vi "ADCP_Update_Data_And_Control_Packets_For_Serial_Port_Reception.vi"(0 "ADCP In":refnum<class "ADCP.lvclass">, 5 "Processed Packet":u8[](array[numeric]), 11 "error in (no error)":errorcluster) -> (4 "ADCP out":refnum<class "ADCP.lvclass">, 6 "Packet Info":T1, 15 "error out":errorcluster)   [LabVIEW 2017, in "ADCP.lvclass"]
uses:
  ADCP.lvclass
  ADCP_Packet_Info.ctl
  ADCP.lvclass/ADCP.ctl
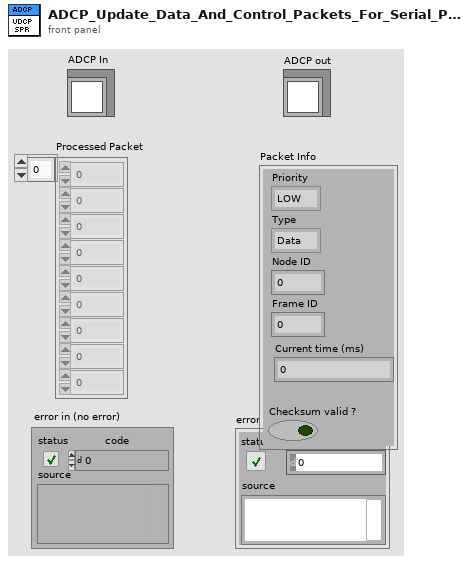
[diagram p1: front panel]
types:
  T1 = typedef "ADCP.lvclass/ADCP_Packet_Info.ctl" = cluster{"Priority":enum16{"LOW", "HIGH"}, "Type":enum16{"Data", "Connection Management", "Remote Request", "Error and status", "INVALID"}, "Node ID":i32, "Frame ID":i32, "Checksum valid ?":bool, "Current time (ms)":u32}
  T2 = enum16{"Data", "Connection Management", "Remote Request", "Error and status", "INVALID"}
  T3 = typedef "ADCP.lvclass/ADCP_Data_Packet_Transmit_Mode.ctl" = enum16{"Disable", "Single", "Cyclic", "Repeat"}
  T4 = cluster{"Parameters":cluster{"Parameter name":string, "Node name":string, "Node ID":u8, "Frame name":string, "Frame ID":u8, "Start bit":u32, "Bit length":u32, "Factor":dbl, "Offset":dbl, "Minimum":dbl, "Maximum":dbl, "Value":string, "Comments":string, "Data_Type":enum16{"BOOL", "UNSIGNED", "SIGNED", "FLOAT32", "ENUM"}, "Enum List":string[]}[], "Priority":enum16{"LOW", "HIGH"}, "Node name":string, "Node ID":u8, "Frame name":string, "Frame ID":u8, "Data":u32, "Raw bytes":u8[], "Processed bytes":u8[], "Tx count":i32, "Last Tx Time":u32, "Tx interval":u32, "Rx count":i32, "Last Rx Time":u32, "Rx interval":u32, "Tx Enable":bool, "Tx mode":T3, "Repeat/Cyclic Tx interval":u32, "Repeat count":u16}[]
  T5 = cluster{"Parameters":cluster{"Parameter name":string, "Node name":string, "Node ID":u8, "Frame name":string, "Frame ID":u8, "Start bit":u32, "Bit length":u32, "Factor":dbl, "Offset":dbl, "Minimum":dbl, "Maximum":dbl, "Value":string, "Comments":string, "Data_Type":enum16{"BOOL", "UNSIGNED", "SIGNED", "FLOAT32", "ENUM"}, "Enum List":string[]}[], "Priority":enum16{"LOW", "HIGH"}, "Node name":string, "Node ID":u8, "Frame name":string, "Frame ID":u8, "Data":u32, "Raw bytes":u8[], "Processed bytes":u8[], "Tx count":i32, "Last Tx Time":u32, "Tx interval":u32, "Rx count":i32, "Last Rx Time":u32, "Rx interval":u32, "Tx Enable":bool, "Tx mode":T3, "Repeat/Cyclic Tx interval":u32, "Repeat count":u16}
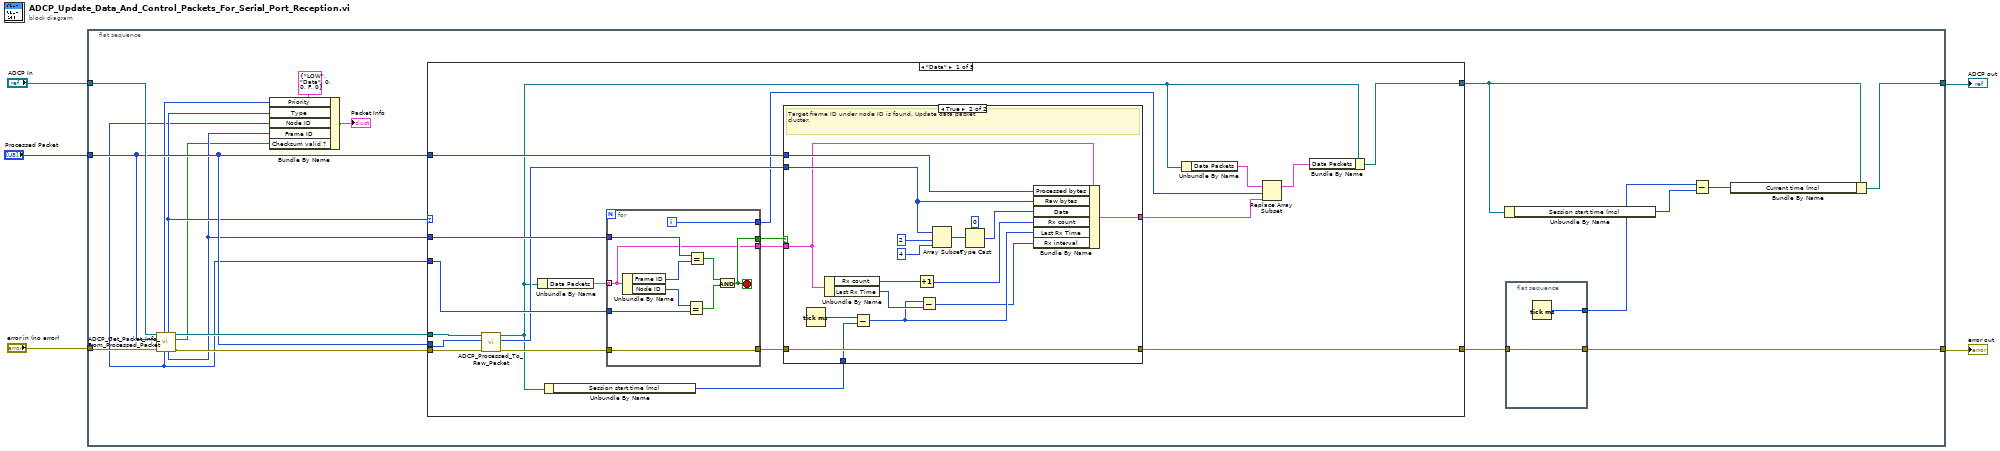
[diagram p0: block diagram]
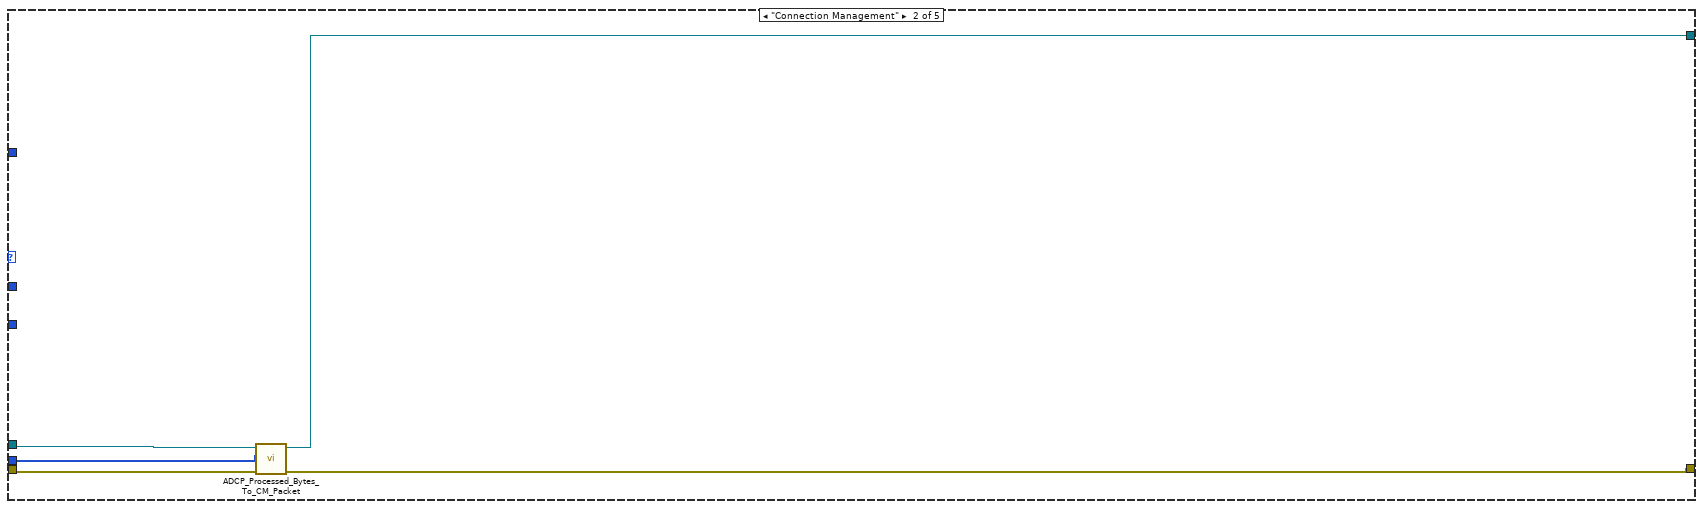
[diagram p3: hidden frame]
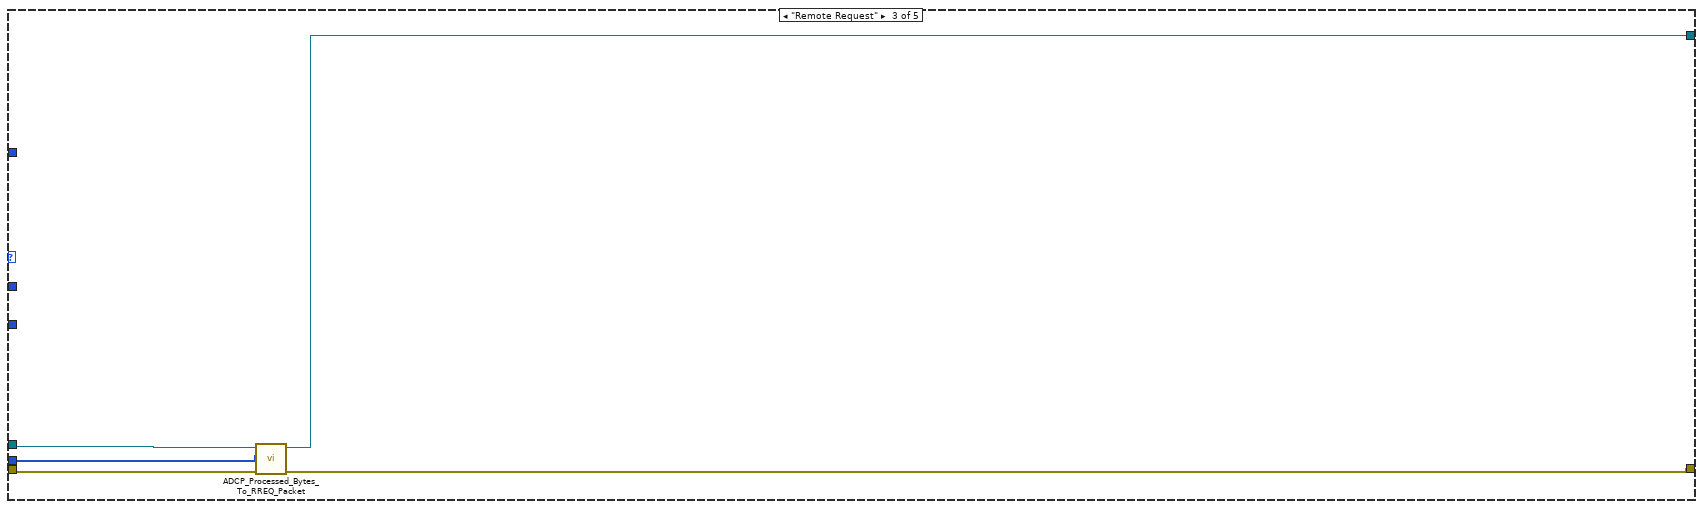
[diagram p4: hidden frame]
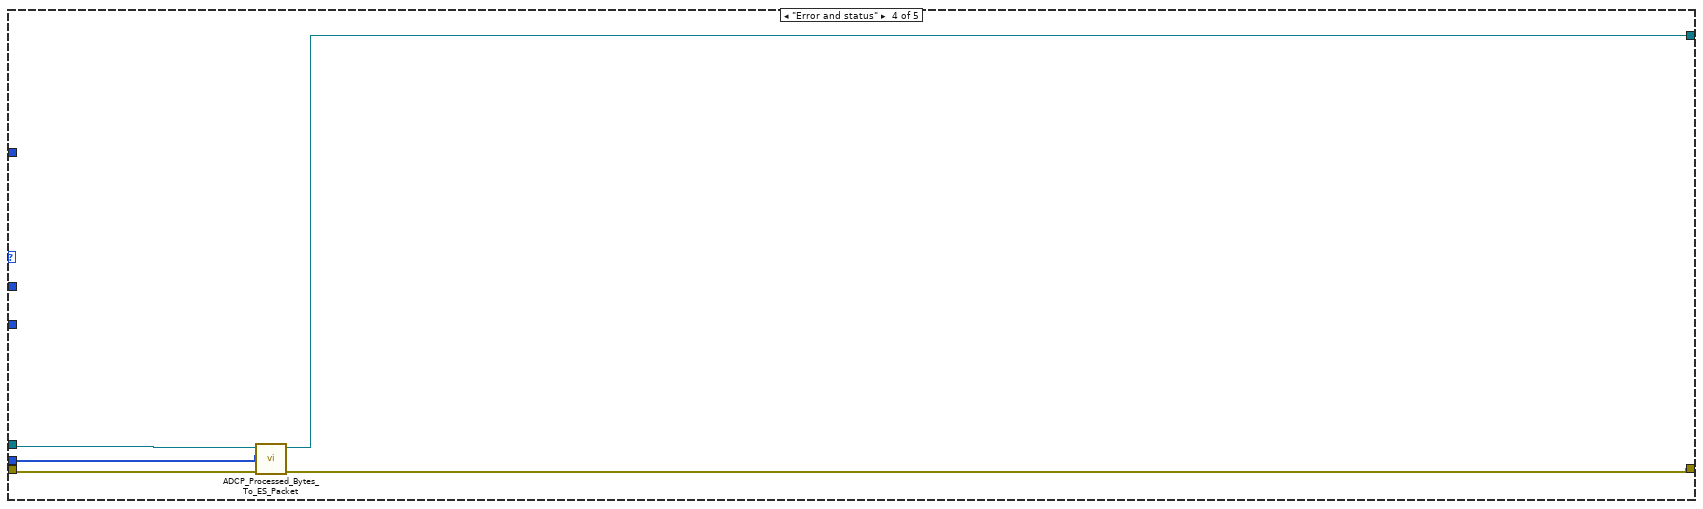
[diagram p5: hidden frame]
diagram:
  n1 = flat-sequence {
    tunnel: "ADCP In" -> [w24]
    tunnel: "Processed Packet" -> [w20]
    tunnel: "error in (no error)" -> [w23]
    tunnel: [w11] -> w1
    tunnel: [w6] -> w2
    frame #0 {
      n2 = call "ADCP_Get_Packet_Info_From_Processed_Packet.vi"("error in (no error)"=w23, "Processed Packet"=w20, "ADCP in"=w24) -> ("error out"=w22:errorcluster, "Checksum Valid ?"=w13:bool, "ADCP out"=w21:refnum<class "ADCP.lvclass">, "Packet frame ID"=w15:u8, "Packet Type"=w17:T2, "Packet node ID"=w16:u8, "Packet_Priority"=w18:enum16{"LOW", "HIGH"})  [unwired: 2 in]
      n3 = Bundle By Name(cluster=T1 {"Priority"=enum."LOW", "Type"=enum."Data", "Node ID"=0, "Frame ID"=0, "Checksum valid ?"=FALSE, "Current time (ms)"=0} ("Packet Info"), "Priority"=w18, "Type"=w17, "Node ID"=w16, "Frame ID"=w15, "Checksum valid ?"=w13) -> (→"Packet Info":T1)
      n4 = case shown="\"Data\"" w17 {
        tunnel: w22 -> [w39 w80 w85 w90 w92]
        tunnel: w21 -> [w37 w79 w84 w89 w91]
        tunnel: w20 -> [w36 w78 w83 w88 _]
        tunnel: w15 -> [w45 _ _ _ _]
        tunnel: w16 -> [w44 _ _ _ _]
        tunnel: w20 -> [w40 _ _ _ _]
        tunnel: [w30 w77 w82 w87 w92] -> w12
        tunnel: [w29 w76 w81 w86 w91] -> w8
        frame "Data" {
          n5 = call "ADCP_Processed_To_Raw_Packet.vi"("error in (no error)"=w39, "Processed Packet"=w36, "ADCP in"=w37) -> ("error out"=w38:errorcluster, "Raw Packet"=w35:u8[], "ADCP out"=w28:refnum<class "ADCP.lvclass">)  [unwired: 6 in]
          n6 = Unbundle By Name(w28) -> ("Data Packets"=w46:T4)
          n7 = Unbundle By Name(w28) -> ("Session start time (ms)"=w27:u32)
          n8 = for {
            tunnel: w38 -> [w71]
            tunnel: w46 -> [w66] mode=indexing
            tunnel: w45 -> [w75]
            tunnel: w44 -> [w72]
            tunnel: [w71] -> w42
            tunnel: [w68] -> w32
            tunnel: [w67] -> w43
            tunnel: [w66] -> w41
            i -> [w68]
            stop <- w67 stop-if-true
            n9 = Unbundle By Name(w66) -> ("Frame ID"=w74:u8, "Node ID"=w73:u8)
            n10 = Equal?(x=w73, y=w72) -> (x = y?=w69:bool)
            n11 = Equal?(x=w75, y=w74) -> (x = y?=w70:bool)
            n12 = And(x=w70, y=w69) -> (x .and. y?=w67:bool)
          }
          n13 = case shown="True" w43 {
            tunnel: w42 -> [w47 w63]
            tunnel: w41 -> [w48 w56]
            tunnel: w40 -> [_ w65]
            tunnel: w35 -> [_ w62]
            tunnel: [w48 w64] -> w33
            tunnel: [w47 w63] -> w30
            tunnel: w27 -> [_ w52]
            frame False {
            }
            frame True {
              # "Target frame ID under node ID is found. Update data packet\ncluster."
              n14 = Tick Count (ms)() -> (millisecond timer value=w53:u32)
              n15 = Unbundle By Name(w56) -> ("Rx count"=w55:i32, "Last Rx Time"=w51:u32)
              n16 = Subtract(x=w53, y=w52) -> (x-y=w50:u32)
              n17 = Increment(x=w55) -> (x+1=w54:i32)
              n18 = Subtract(x=w50, y=w51) -> (x-y=w49:u32)
              n19 = Array Subset(array=w62, index=2, length=4) -> (w59:u8[])
              n20 = Type Cast(type=u32 0, x=w59) -> (*(type *) &x=w57:u32)
              n21 = Bundle By Name(cluster=w56, "Processed bytes"=w65, "Raw bytes"=w62, "Data"=w57, "Rx count"=w54, "Last Rx Time"=w50, "Rx interval"=w49) -> (w64:T5)
            }
          }
          n22 = Unbundle By Name(w28) -> ("Data Packets"=w34:T4)
          n23 = Replace Array Subset(array=w34, new element=w33, index=w32) -> (w31:T4)
          n24 = Bundle By Name(cluster=w28, "Data Packets"=w31) -> (w29:refnum<class "ADCP.lvclass">)
        }
        frame "Connection Management" {
          n25 = call "ADCP_Processed_Bytes_To_CM_Packet.vi"("error in (no error)"=w80, "Processed Packet Bytes"=w78, "ADCP In"=w79) -> ("error out"=w77:errorcluster, "ADCP out"=w76:refnum<class "ADCP.lvclass">)  [unwired: 6 in, 1 out]
        }
        frame "Remote Request" {
          n26 = call "ADCP_Processed_Bytes_To_RREQ_Packet.vi"("error in (no error)"=w85, "Processed Packet Bytes"=w83, "ADCP In"=w84) -> ("error out"=w82:errorcluster, "ADCP Out"=w81:refnum<class "ADCP.lvclass">)  [unwired: 6 in, 1 out]
        }
        frame "Error and status" {
          n27 = call "ADCP_Processed_Bytes_To_ES_Packet.vi"("error in (no error)"=w90, "Processed Packet Bytes"=w88, "ADCP In"=w89) -> ("error out"=w87:errorcluster, "ADCP Out"=w86:refnum<class "ADCP.lvclass">)  [unwired: 6 in, 1 out]
        }
        frame "INVALID", Default {
        }
      }
      n28 = Unbundle By Name(w8) -> ("Session start time (ms)"=w10:u32)
      n29 = flat-sequence {
        tunnel: w12 -> [w26]
        tunnel: [w26] -> w11
        tunnel: [w25] -> w9
        frame #0 {
          n30 = Tick Count (ms)() -> (millisecond timer value=w25:u32)
        }
      }
      n31 = Subtract(x=w9, y=w10) -> (x-y=w7:u32)
      n32 = Bundle By Name(cluster=w8, "Current time (ms)"=w7) -> (w6:refnum<class "ADCP.lvclass">)
    }
  }
  "ADCP out" <- w2
  "error out" <- w1
